vi "set up acquisition parameters.vi"(6 "error in (no error)":errorcluster, 7 "Acquisition Parameters":T2={"Readout Mode"=enum."Full Vertical Binning", "Set Acquisition Mode"=enum."(do nothing)", "Trigger Mode"=enum."Internal", "Exposure Time (s)"=0.0, "Accumulation Cycle (s)"=0.0, "Kinetic Cycle Time (s)"=0.0, "Number of Kinetics"=0, "Number of Accumulations"=0, "Set VS Speed"=0, "Pixel Rate"=enum."Standard CCD 3 Mhz 14 bits", "V Shift Amplitude"=enum."+1", "Preamp Gain"=enum."1.0"}, 8 "Image Size":T1) -> (0 "error out":errorcluster, 1 "Kinetics":dbl format="%#_13g", 2 "Accumulation":dbl format="%#_13g", 3 "Exposure":dbl format="%#_13g", 9 "High Capacity?":bool)   [LabVIEW 2014]
uses:
  Initilize Globals.vi
  lib/Andorlib/atmcd32d.dll
  lib/Andorlib/atmcd32d.lvlib
panel:
  in  "EM CCD Gain":u16(slide)=230 scale=0.01..255.0
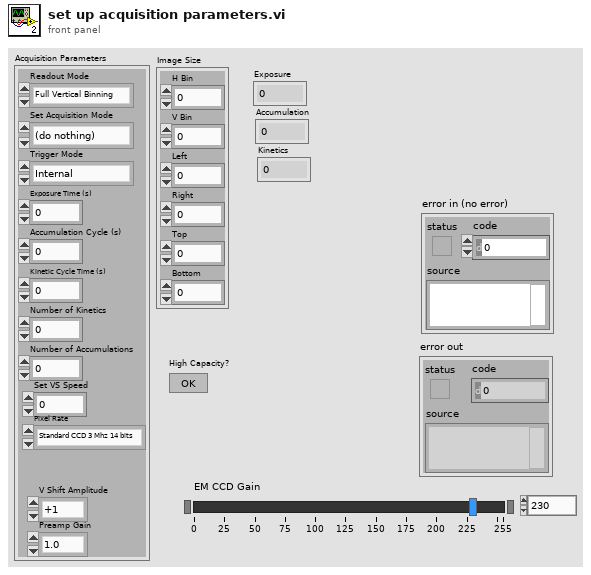
[diagram p1: front panel]
types:
  T1 = cluster{"H Bin":dbl, "V Bin":dbl, "Left":dbl, "Right":dbl, "Top":dbl, "Bottom":dbl}
  T2 = cluster{"Readout Mode":enum16{"Full Vertical Binning", "Multi-Track", "Random-Track", "Single-Track", "Image"}, "Set Acquisition Mode":enum16{"(do nothing)", "Single Scan", "Accumulate", "Kinetics", "Fast Kinetics", "Run till abort"}, "Trigger Mode":enum16{"Internal", "External"}, "Exposure Time (s)":dbl, "Accumulation Cycle (s)":dbl, "Kinetic Cycle Time (s)":dbl, "Number of Kinetics":i32, "Number of Accumulations":i32, "Set VS Speed":i32, "Pixel Rate":enum16{"EM CCD 10 Mhz 14 bits", "EM CCD 5 Mhz 14 bits", "EM CCD 3 Mhz 14 bits", "EM CCD 1 Mhz 16 bits", "Standard CCD 3 Mhz 14 bits", "Standard CCD 1 Mhz 16 bits"}, "V Shift Amplitude":enum16{"normal", "+1", "+2", "+3", "+4"}, "Preamp Gain":enum16{"1.0", "2.4", "5.0"}}
  T3 = cluster{"Adc Channel":i32, "H Shift Setting":i32, "EM on?":bool}[]
  T4 = enum16{"Full Vertical Binning", "Multi-Track", "Random-Track", "Single-Track", "Image"}
  T5 = enum16{"(do nothing)", "Single Scan", "Accumulate", "Kinetics", "Fast Kinetics", "Run till abort"}
  T6 = enum16{"EM CCD 10 Mhz 14 bits", "EM CCD 5 Mhz 14 bits", "EM CCD 3 Mhz 14 bits", "EM CCD 1 Mhz 16 bits", "Standard CCD 3 Mhz 14 bits", "Standard CCD 1 Mhz 16 bits"}
  T7 = cluster{"Adc Channel":i32, "H Shift Setting":i32, "EM on?":bool}
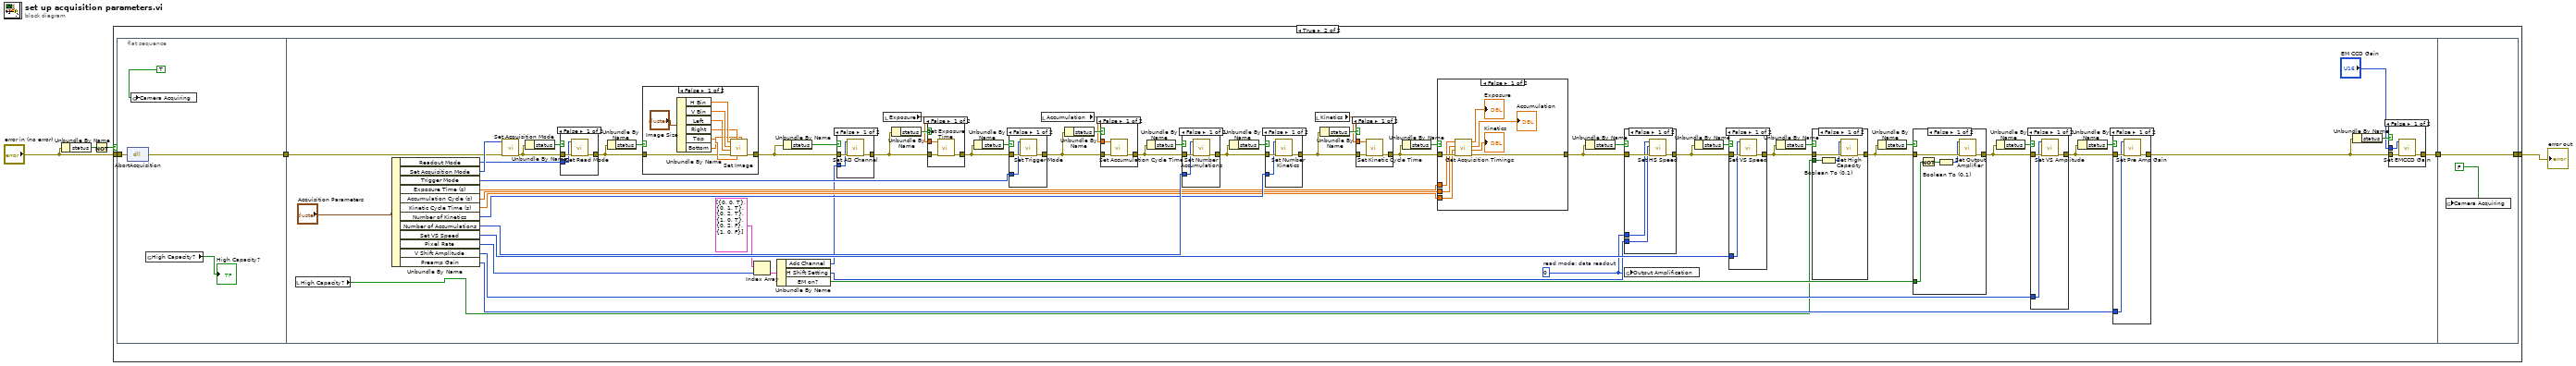
[diagram p0: block diagram]
diagram:
  n1 = Unbundle By Name("error in (no error)") -> ("status"=w4:bool)
  n2 = Not(x=w4) -> (.not. x?=w3:bool)
  n3 = case shown="True" w3 {
    tunnel: "error in (no error)" -> [w5 w8]
    tunnel: [w5 w7] -> w1
    frame False {
    }
    frame True {
      n4 = flat-sequence {
        tunnel: [w12] -> w9
        tunnel: w8 -> [w13]
        tunnel: w9 -> [w18]
        tunnel: [w17] -> w6
        tunnel: [w158] -> w7
        tunnel: w6 -> [w158]
        frame #0 {
          n5 = dll-call lib="C:/Users/Bakir/Desktop/LabFiles/Testing/lib/Andorlib/ATMCD32D.DLL" fn="AbortAcquisition" label="Call Library Function\nAbort"(error in=w13) -> (error out=w12:errorcluster)  [unwired: 2 in, 2 out]
          n6 = global write "Initilize Globals.vi" "Camera Acquiring"(TRUE) -> ()
          n7 = global read "Initilize Globals.vi" "High Capacity?"() -> (→"High Capacity?":bool)
        }
        frame #1 {
          w32 = 0  # read mode: data readout
          n8 = local read "High Capacity?"() -> (w15:bool)
          n9 = Unbundle By Name("Acquisition Parameters") -> ("Readout Mode"=w53:T4, "Set Acquisition Mode"=w54:T5, "Trigger Mode"=w52:enum16{"Internal", "External"}, "Exposure Time (s)"=w47:dbl, "Accumulation Cycle (s)"=w48:dbl, "Kinetic Cycle Time (s)"=w46:dbl, "Number of Kinetics"=w50:i32, "Number of Accumulations"=w51:i32, "Set VS Speed"=w49:i32, "Pixel Rate"=w39:T6, "V Shift Amplitude"=w21:enum16{"normal", "+1", "+2", "+3", "+4"}, "Preamp Gain"=w20:enum16{"1.0", "2.4", "5.0"})
          n10 = call "Set Acquisition Mode.vi"("error in (no error)"=w18, "mode"=w54) -> ("error out"=w56:errorcluster)  [unwired: 8 in, 1 out]
          n11 = Unbundle By Name(w56) -> ("status"=w57:bool)
          n12 = case shown="False" w57 {
            tunnel: w56 -> [w113 w114]
            tunnel: [w112 w114] -> w41
            tunnel: w53 -> [w111 _]
            frame False {
              n13 = call "Set Read Mode.vi"("error in (no error)"=w113, "mode"=w111) -> ("error out"=w112:errorcluster)  [unwired: 8 in, 1 out]
            }
            frame True {
            }
          }
          n14 = Unbundle By Name(w41) -> ("status"=w42:bool)
          n15 = case shown="False" w42 {
            tunnel: w41 -> [w102 w110]
            tunnel: [w101 w110] -> w35
            frame False {
              n16 = Unbundle By Name("Image Size") -> ("H Bin"=w108:dbl, "V Bin"=w107:dbl, "Left"=w106:dbl, "Right"=w105:dbl, "Top"=w104:dbl, "Bottom"=w103:dbl)
              n17 = call "Set Image.vi"("vend"=w103, "vstart"=w104, "hend"=w105, "error in (no error)"=w102, "hstart"=w106, "vbin"=w107, "hbin"=w108) -> ("error out"=w101:errorcluster)  [unwired: 3 in, 1 out]
            }
            frame True {
            }
          }
          n18 = Index Array(array=T3 [{"Adc Channel"=0, "H Shift Setting"=0, "EM on?"=TRUE}, {"Adc Channel"=0, "H Shift Setting"=1, "EM on?"=TRUE}, {"Adc Channel"=0, "H Shift Setting"=2, "EM on?"=TRUE}, {"Adc Channel"=1, "H Shift Setting"=0, "EM on?"=TRUE}, {"Adc Channel"=0, "H Shift Setting"=2, "EM on?"=FALSE}, {"Adc Channel"=1, "H Shift Setting"=0, "EM on?"=FALSE}], index=w39) -> (element=w38:T7)
          n19 = Unbundle By Name(w38) -> ("Adc Channel"=w34:i32, "H Shift Setting"=w33:i32, "EM on?"=w22:bool)
          n20 = Unbundle By Name(w35) -> ("status"=w37:bool)
          n21 = case shown="False" w37 {
            tunnel: [w98 w100] -> w36
            tunnel: w35 -> [w99 w100]
            tunnel: w34 -> [w97 _]
            frame False {
              n22 = call "Set AD Channel.vi"("error in (no error)"=w99, "channel"=w97) -> ("error out"=w98:errorcluster)  [unwired: 8 in, 1 out]
            }
            frame True {
            }
          }
          n23 = local read "Exposure"() -> (w45:dbl)
          n24 = Unbundle By Name(w36) -> ("status"=w55:bool)
          n25 = case shown="False" w55 {
            tunnel: w36 -> [w155 w156]
            tunnel: [w154 w156] -> w65
            tunnel: w45 -> [w153 _]
            frame False {
              n26 = call "Set Exposure Time.vi"("error in (no error)"=w155, "time"=w153) -> ("error out"=w154:errorcluster)  [unwired: 8 in, 1 out]
            }
            frame True {
            }
          }
          n27 = Unbundle By Name(w65) -> ("status"=w73:bool)
          n28 = case shown="False" w73 {
            tunnel: w65 -> [w151 w152]
            tunnel: [w150 w152] -> w64
            tunnel: w52 -> [w149 _]
            frame False {
              n29 = call "Set Trigger Mode.vi"("error in (no error)"=w151, "mode"=w149) -> ("error out"=w150:errorcluster)  [unwired: 8 in, 1 out]
            }
            frame True {
            }
          }
          n30 = local read "Accumulation"() -> (w44:dbl)
          n31 = Unbundle By Name(w64) -> ("status"=w72:bool)
          n32 = case shown="False" w72 {
            tunnel: w64 -> [w147 w148]
            tunnel: [w146 w148] -> w63
            tunnel: w44 -> [w145 _]
            frame False {
              n33 = call "Set Accumulation Cycle Time.vi"("error in (no error)"=w147, "time"=w145) -> ("error out"=w146:errorcluster)  [unwired: 8 in, 1 out]
            }
            frame True {
            }
          }
          n34 = Unbundle By Name(w63) -> ("status"=w71:bool)
          n35 = case shown="False" w71 {
            tunnel: w63 -> [w143 w144]
            tunnel: [w142 w144] -> w62
            tunnel: w51 -> [w141 _]
            frame False {
              n36 = call "Set Number Accumulations.vi"("error in (no error)"=w143, "number"=w141) -> ("error out"=w142:errorcluster)  [unwired: 8 in, 1 out]
            }
            frame True {
            }
          }
          n37 = Unbundle By Name(w62) -> ("status"=w70:bool)
          n38 = case shown="False" w70 {
            tunnel: w62 -> [w139 w140]
            tunnel: [w138 w140] -> w61
            tunnel: w50 -> [w137 _]
            frame False {
              n39 = call "Set Number Kinetics.vi"("error in (no error)"=w139, "number"=w137) -> ("error out"=w138:errorcluster)  [unwired: 8 in, 1 out]
            }
            frame True {
            }
          }
          n40 = local read "Kinetics"() -> (w43:dbl)
          n41 = Unbundle By Name(w61) -> ("status"=w69:bool)
          n42 = case shown="False" w69 {
            tunnel: w61 -> [w135 w136]
            tunnel: [w134 w136] -> w60
            tunnel: w43 -> [w133 _]
            frame False {
              n43 = call "Set Kinetic Cycle Time.vi"("error in (no error)"=w135, "time"=w133) -> ("error out"=w134:errorcluster)  [unwired: 8 in, 1 out]
            }
            frame True {
            }
          }
          n44 = Unbundle By Name(w60) -> ("status"=w68:bool)
          n45 = case shown="False" w68 {
            tunnel: w60 -> [w131 w132]
            tunnel: [w130 w132] -> w59
            tunnel: w48 -> [w129 _]
            tunnel: w47 -> [w128 _]
            tunnel: w46 -> [w127 _]
            frame False {
              n46 = call "Get Acquisition Timings.vi"("error in (no error)"=w131, "kinetic"=w127, "accumulate"=w129, "exposure"=w128) -> ("error out"=w130:errorcluster, "kinetic out"=→"Kinetics":sgl, "accumulate out"=→"Accumulation":sgl, "exposure out"=→"Exposure":sgl)  [unwired: 3 in, 1 out]
            }
            frame True {
            }
          }
          n47 = Unbundle By Name(w59) -> ("status"=w67:bool)
          n48 = case shown="False" w67 {
            tunnel: w59 -> [w122 w123]
            tunnel: [w121 w123] -> w58
            tunnel: w33 -> [w120 _]
            tunnel: w32 -> [w119 _]
            frame False {
              n49 = call "Set HS Speed.vi"("error in (no error)"=w122, "index"=w120, "typ"=w119) -> ("error out"=w121:errorcluster)  [unwired: 7 in, 1 out]
            }
            frame True {
            }
          }
          n50 = global write "Initilize Globals.vi" "Output Amplification"(w32) -> ()
          n51 = Unbundle By Name(w58) -> ("status"=w66:bool)
          n52 = case shown="False" w66 {
            tunnel: w58 -> [w117 w118]
            tunnel: [w116 w118] -> w26
            tunnel: w49 -> [w115 _]
            frame False {
              n53 = call "Set VS Speed.vi"("error in (no error)"=w117, "index"=w115) -> ("error out"=w116:errorcluster)  [unwired: 8 in, 1 out]
            }
            frame True {
            }
          }
          n54 = Unbundle By Name(w26) -> ("status"=w31:bool)
          n55 = case shown="False" w31 {
            tunnel: [w94 w96] -> w25
            tunnel: w26 -> [w95 w96]
            tunnel: w15 -> [w92 _]
            frame False {
              n56 = Boolean To (0,1)(Boolean=w92) -> (0, 1=w93:i16)
              n57 = call "Set High Capacity.vi"("error in (no error)"=w95, "state"=w93) -> ("error out"=w94:errorcluster)  [unwired: 8 in, 1 out]
            }
            frame True {
            }
          }
          n58 = Unbundle By Name(w25) -> ("status"=w30:bool)
          n59 = case shown="False" w30 {
            tunnel: [w89 w91] -> w24
            tunnel: w25 -> [w90 w91]
            tunnel: w22 -> [w86 _]
            frame False {
              n60 = Not(x=w86) -> (.not. x?=w87:bool)
              n61 = Boolean To (0,1)(Boolean=w87) -> (0, 1=w88:i16)
              n62 = call "Set Output Amplifier.vi"("error in (no error)"=w90, "typ"=w88) -> ("error out"=w89:errorcluster)  [unwired: 8 in, 1 out]
            }
            frame True {
            }
          }
          n63 = Unbundle By Name(w24) -> ("status"=w29:bool)
          n64 = case shown="False" w29 {
            tunnel: [w83 w85] -> w23
            tunnel: w24 -> [w84 w85]
            tunnel: w21 -> [w82 _]
            frame False {
              n65 = call "Set VS Amplitude.vi"("error in (no error)"=w84, "index"=w82) -> ("error out"=w83:errorcluster)  [unwired: 8 in, 1 out]
            }
            frame True {
            }
          }
          n66 = Unbundle By Name(w23) -> ("status"=w28:bool)
          n67 = case shown="False" w28 {
            tunnel: [w79 w81] -> w14
            tunnel: w23 -> [w80 w81]
            tunnel: w20 -> [w78 _]
            frame False {
              n68 = call "Set Pre Amp Gain.vi"("error in (no error)"=w80, "index"=w78) -> ("error out"=w79:errorcluster)  [unwired: 8 in, 1 out]
            }
            frame True {
            }
          }
          n69 = Unbundle By Name(w14) -> ("status"=w27:bool)
          n70 = case shown="False" w27 {
            tunnel: [w75 w77] -> w17
            tunnel: w14 -> [w76 w77]
            tunnel: "EM CCD Gain" -> [w74 _]
            frame False {
              n71 = call "Set EMCCD Gain.vi"("error in (no error)"=w76, "gain"=w74) -> ("error out"=w75:errorcluster)  [unwired: 8 in, 1 out]
            }
            frame True {
            }
          }
        }
        frame #2 {
          n72 = global write "Initilize Globals.vi" "Camera Acquiring"(FALSE) -> ()
        }
      }
    }
  }
  "error out" <- w1
